vi "Aging System Summary.vi"(2 "System":string) -> ()   [LabVIEW 2023]
uses:
  <vilib>/Utility/file.llb/Read Delimited Spreadsheet (string).vi
panel:
  out "SystemMessage":string
  in  "OK":bool
  out "ActivePositions":string
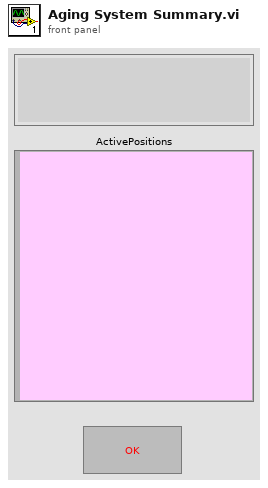
[diagram p1: front panel]
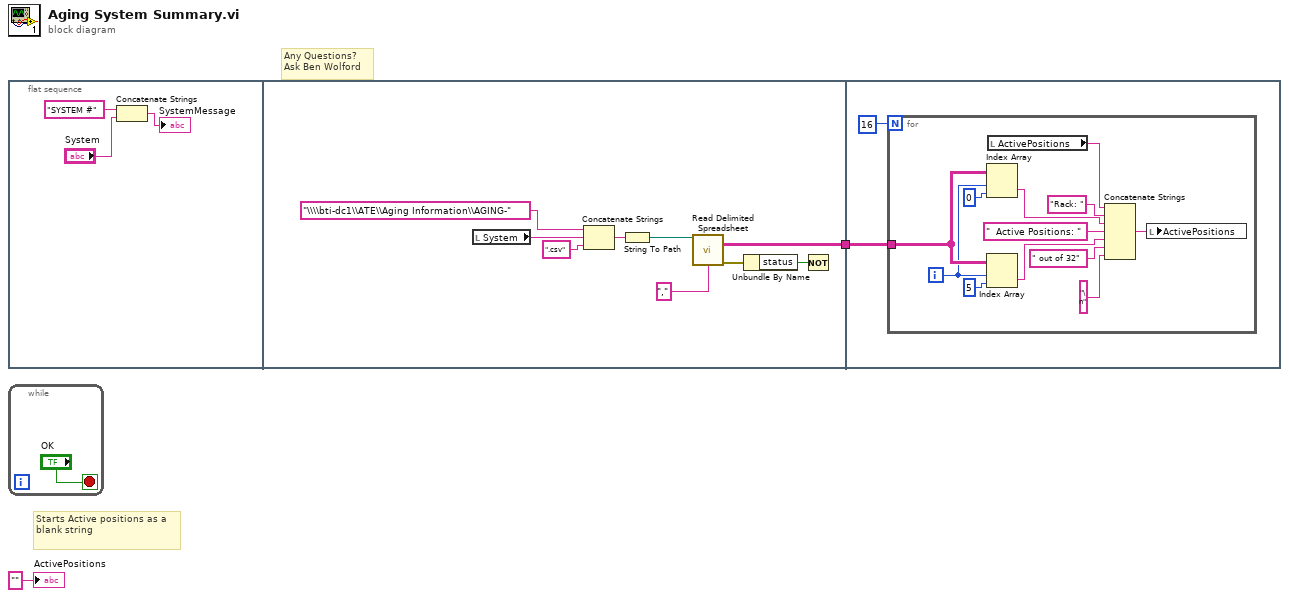
[diagram p0: block diagram]
diagram:
  # "Starts Active positions as a blank string"
  # "Any Questions?\nAsk Ben Wolford"
  n1 = flat-sequence {
    tunnel: [w10] -> w1
    tunnel: w1 -> [w16]
    frame #0 {
      n2 = Concatenate Strings("SYSTEM #" ("string"), "System") -> (→"SystemMessage":string)
    }
    frame #1 {
      n3 = local read "System"() -> (w8:string)
      n4 = Concatenate Strings("\\\\bti-dc1\\ATE\\Aging Information\\AGING-" ("string"), w8, ".csv" ("string")) -> (w7:string)
      n5 = String To Path(string=w7) -> (path=w13:path)
      n6 = call-poly <vilib>:"Read Delimited Spreadsheet.vi"("file path (dialog if empty)"=w13, "delimiter (\\t)"="," ("delimiter (\\t)")) -> ("all rows"=w10:string[][], "error out"=w12:errorcluster)  [unwired: 8 in, 4 out]
      n7 = Unbundle By Name(w12) -> ("status"=w14:bool)
      n8 = Not(x=w14) -> ()  [unwired: 1 out]
    }
    frame #2 {
      n9 = for {
        N: 16 -> [_]
        tunnel: w16 -> [w22]
        i -> [w21]
        n10 = Index Array(array=w22, index (row)=w21, index (col)=0 ("disabled index (col)")) -> (element=w18:string)
        n11 = Index Array(array=w22, index (row)=w21, index (col)=5 ("disabled index (col)")) -> (element=w17:string)
        n12 = local read "ActivePositions"() -> (w28:string)
        n13 = Concatenate Strings(w28, "Rack: " ("string"), w18, "  Active Positions: " ("string"), w17, " out of 32" ("string"), "\n" ("string")) -> (w27:string)
        n14 = local write "ActivePositions"(w27) -> ()
      }
    }
  }
  n15 = while {
    stop <- "OK" stop-if-true
  }
  "ActivePositions" <- "" ("ActivePositions")
